vi "Meas_Fast_FID_Bkgnd.vi"(3 "Mode":T5, 5 "Traverse line In":T2 {"Row Duration (mins)" format="%#.1f"; "Row No" min=0; "Trace Gas Concentration (%)" min=0.0 format="%#.2f"; "Emission Rate (l/min)" format="%#.2f"; "Tunnel Speed" format="%#.2f"; "Start X" format="%#.2f"; "Start Y" format="%#.2f"; "Start Z" format="%#.2f"; "End X" format="%#.2f"; "End Y" format="%#.2f"; "End Z" format="%#.2f"; "Averaging time (min)" min=0.0 format="%#.2f"}) -> (0 "Error Message":string, 1 "Status":T1, 2 "Traverse line Out":T2 {"Row Duration (mins)" format="%#.1f"; "Row No" min=0; "Trace Gas Concentration (%)" min=0.0 format="%#.2f"; "Emission Rate (l/min)" format="%#.2f"; "Tunnel Speed" format="%#.2f"; "Start X" format="%#.2f"; "Start Y" format="%#.2f"; "Start Z" format="%#.2f"; "End X" format="%#.2f"; "End Y" format="%#.2f"; "End Z" format="%#.2f"; "Averaging time (min)" min=0.0 format="%#.2f"})   [LabVIEW 2012]
uses:
  Gen Trav/Traverse_cluster.ctl
  Gen Trav/Spacing.ctl
  Controls/Multi_run_mode.ctl
  Controls/User_Specific_mode.ctl
  Gen Trav/Multi_Run_Status.ctl
  Gen Trav/Trav_mode.ctl
  File/Setup_Filetype.ctl
  Controls/Setup.ctl
  Controls/Save_Data.ctl
  Globals/Trav_pos_global.vi
  Globals/Preference_global.vi
panel:
  out "Initial Trav Pos":dbl[](array[numeric]) format="%#.2f"
  # "X           Y            Z"
  # "Start"
  # "End"
  # "X           Y            Z"
  # "Start"
  # "End"
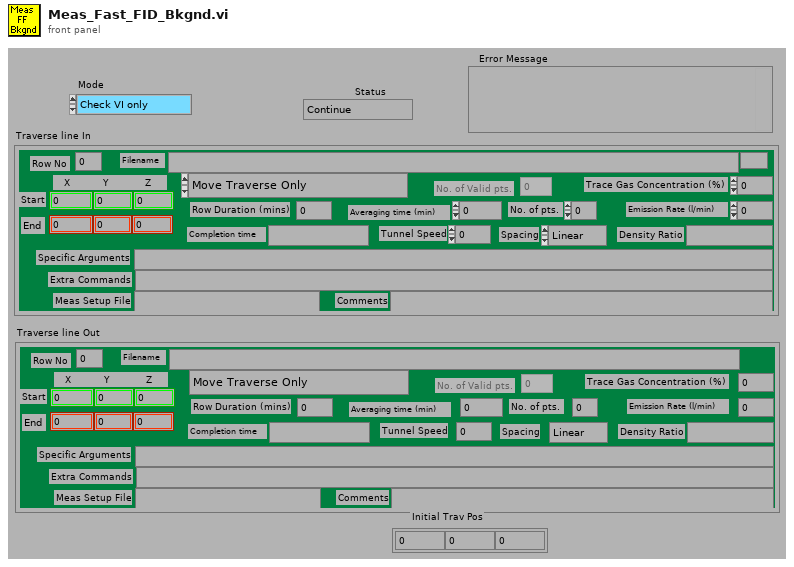
[diagram p1: front panel]
types:
  T1 = typedef "Multi_Run_Status.ctl" = enum16{"Continue", "Jump to Next Point", "Jump to Next Row", "Jump To Fall Back", "Terminate Run"}
  T2 = typedef "Traverse_cluster.ctl" = cluster{"Start X":dbl, "Start Y":dbl, "Start Z":dbl, "End X":dbl, "End Y":dbl, "End Z":dbl, "No. of pts.":i32, "Spacing":T3, "Filename":path, "Tunnel Speed":dbl, "Averaging time (min)":dbl, "Extra Commands":string, "Specific Arguments":string, "Emission Rate (l/min)":dbl, "Trace Gas Concentration (%)":dbl, "Density Ratio":string, "Comments":string, "Row No":i32, "Row Type Selector":T4, "Completion time":string, "Row Duration (mins)":dbl, "No. of Valid pts.":i32, "Meas Setup File":string}
  T3 = typedef "Spacing.ctl" = enum16{"Linear", "Log", "Gauss", "Specified", "N/A"}
  T4 = typedef "Multi_run_mode.ctl" = enum16{"Move Traverse Only", "Set Tunnel Speed Only", "Set Source Only", "Set Measurement Conditions", "Single Measurement", "Vertical Profile", "Lateral Profile", "Longitudinal Profile", "Explore Volume", "Multi-Axis Profile", "Auto Calibrate", "Meas Fast FID Bkgnd", "Check Beam Power", "Scanning Valve Measurement", "Run VI Named:", "Set ADAM Ch", "Wait (minutes)", "Send Message", "Synchronize With:", "Fall Back to this Row", "Turn Off Row Repeating", "Blank Row", "Traverse 3D Volume"}
  T5 = typedef "User_Specific_mode.ctl" = enum16{"Check VI only", "Run VI"}
  T6 = typedef "Tunnel_Coordinates.ctl" = enum16{"Work in Tunnel Coordinates", "Work in Model Coordinates"}
  T7 = typedef "Trav_mode.ctl" = enum16{"Move traverse", "Read traverse position", "Teach Position"}
  T8 = typedef "Setup_Filetype.ctl" = enum16{"Measurement Setups", "Calibration Setups", "General", "Results File Plotter Setups", "Speed Calib Tweaks"}
  T9 = typedef "Save_Data.ctl" = enum16{"Save No Data", "Save Data"}
  T10 = typedef "Setup.ctl" = enum16{"Run Program", "Show Setup", "Save Current Setup", "Setup Front Panel"}
  T11 = typedef "Status_Cluster.ctl" = cluster{"Status":T1, "Error Type":string, "Error Description":string}
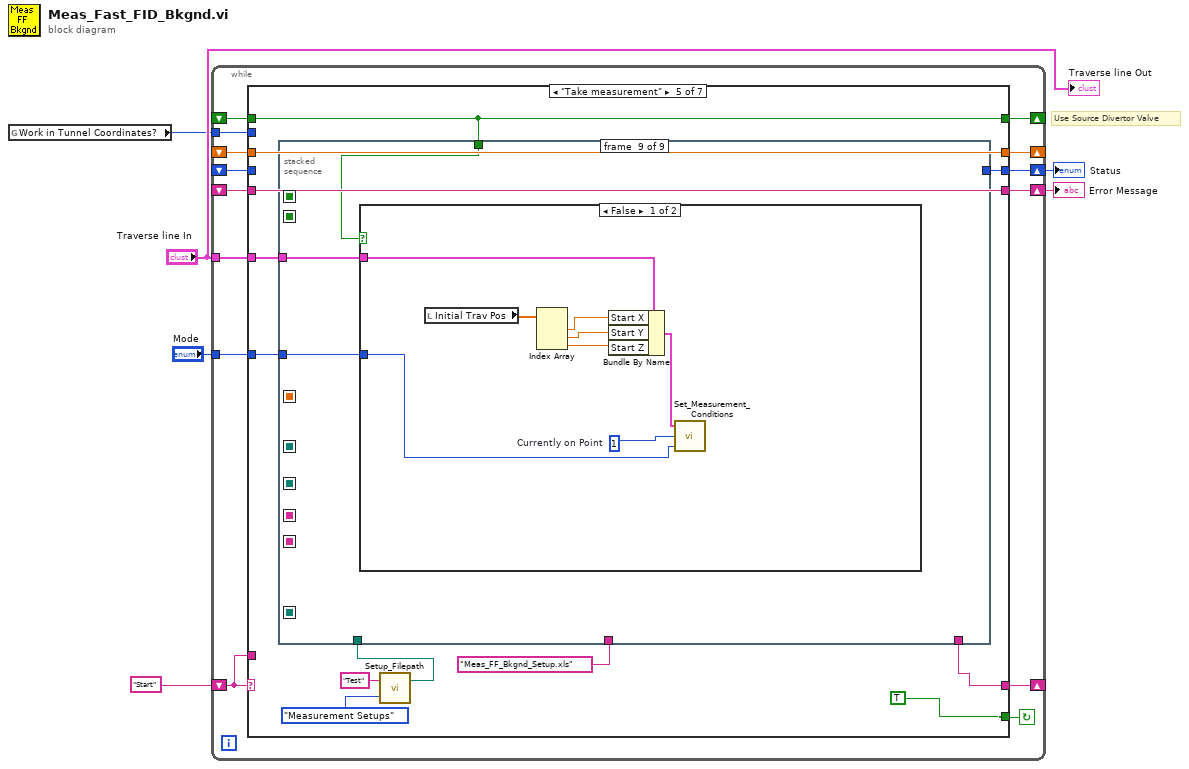
[diagram p0: block diagram]
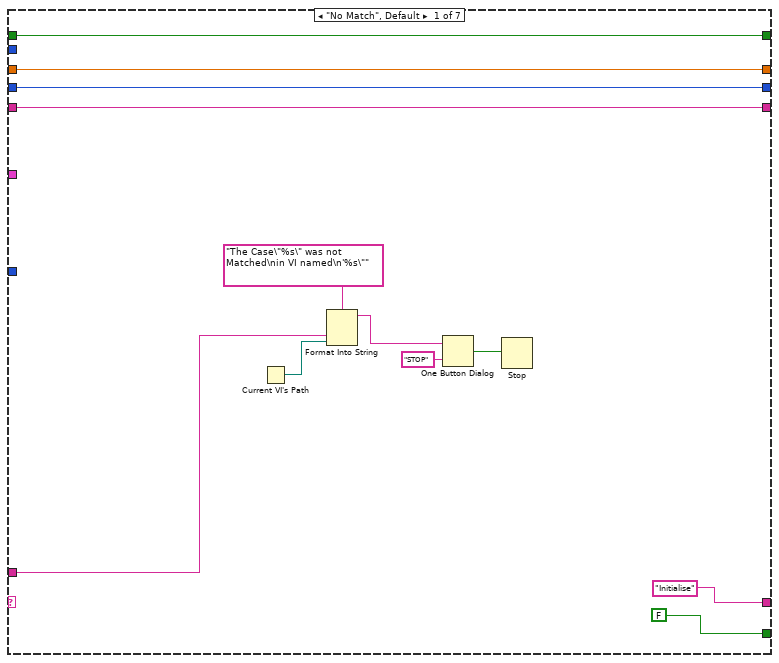
[diagram p2: hidden frame]
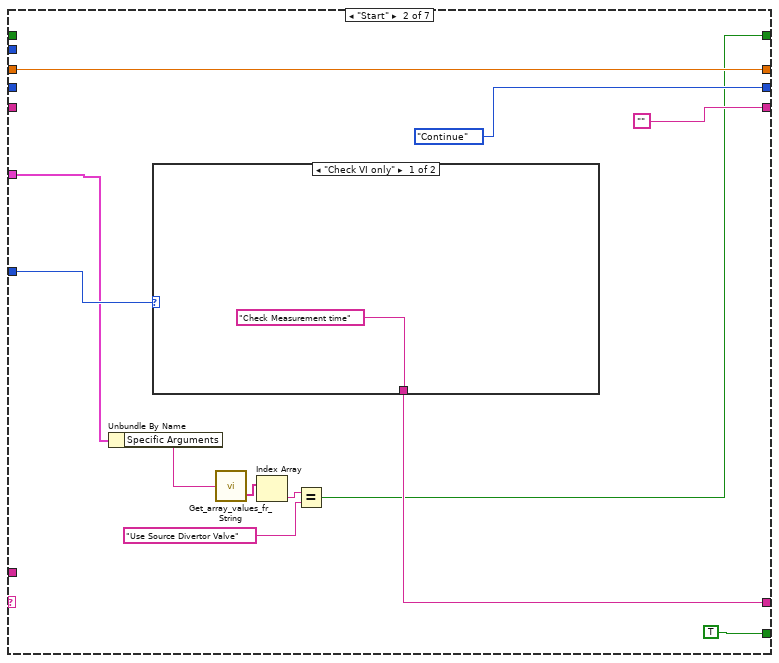
[diagram p3: hidden frame]
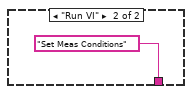
[diagram p4: hidden frame]
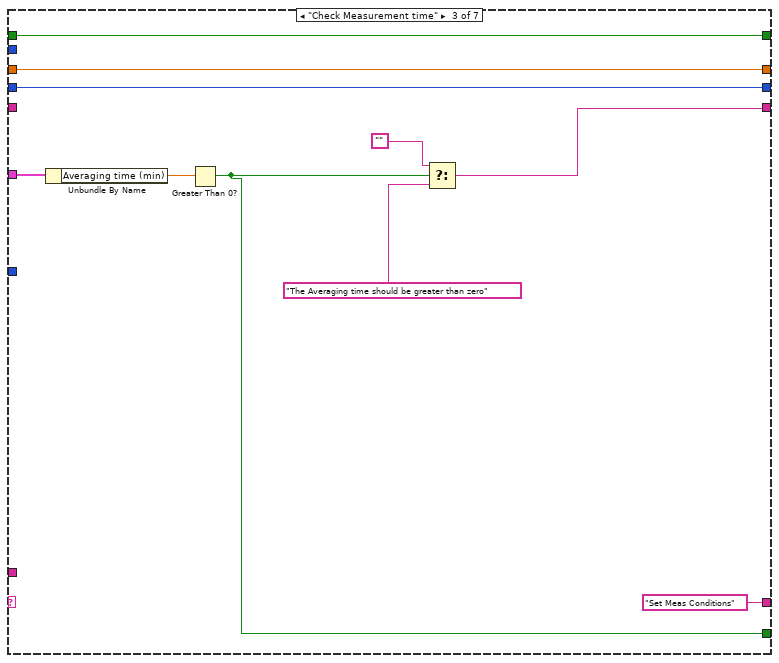
[diagram p5: hidden frame]
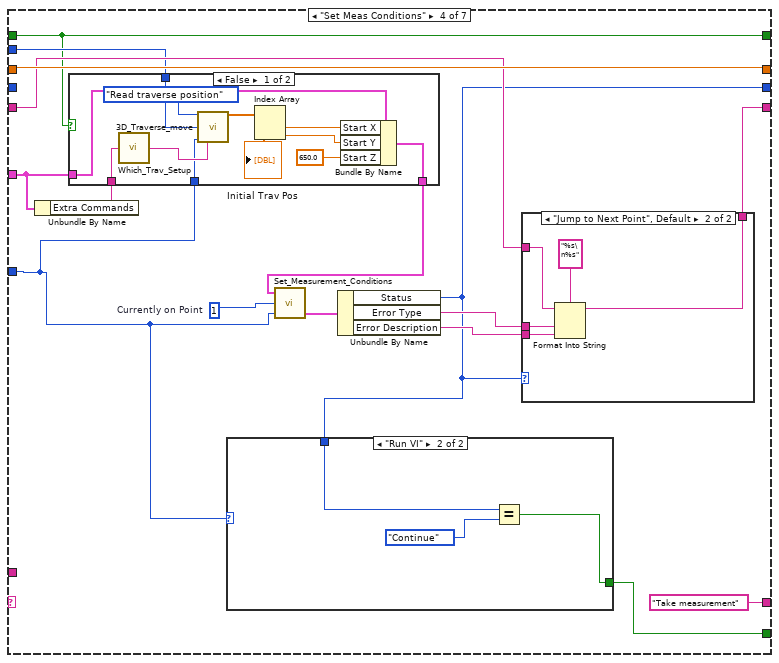
[diagram p6: hidden frame]
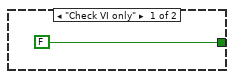
[diagram p9: hidden frame]
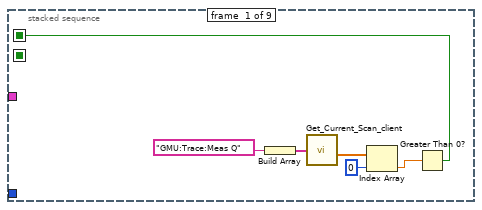
[diagram p10: hidden frame]
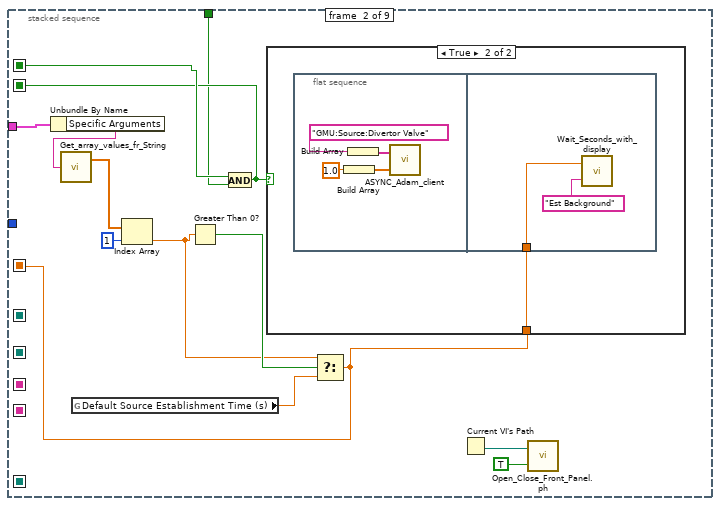
[diagram p11: hidden frame]
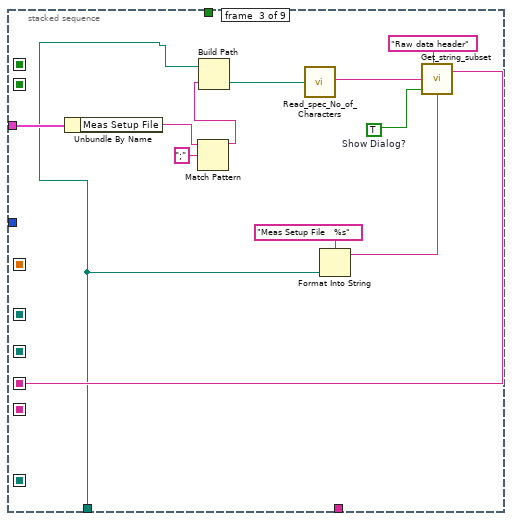
[diagram p13: hidden frame]
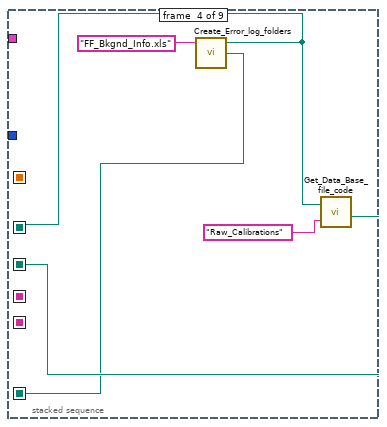
[diagram p14: hidden frame]
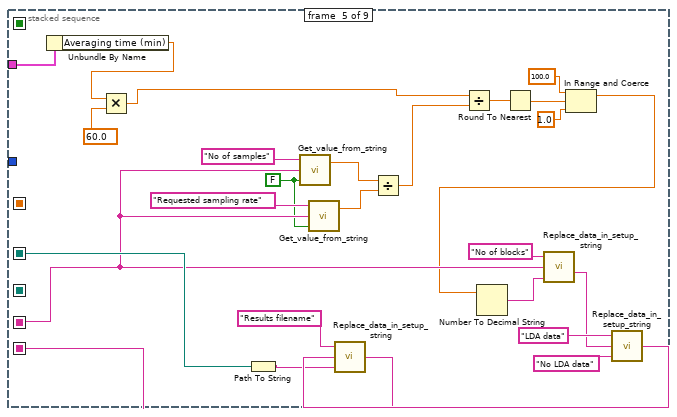
[diagram p15: hidden frame]
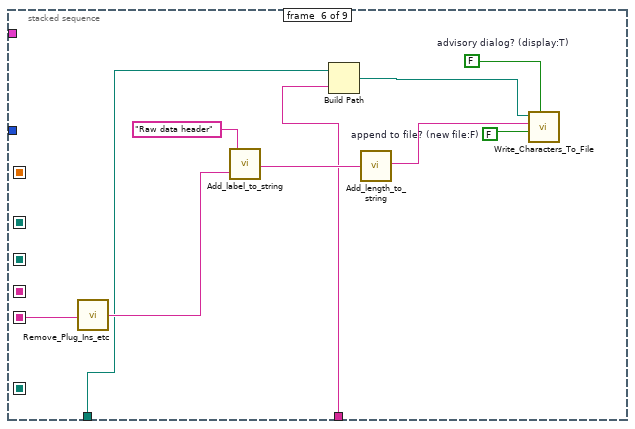
[diagram p16: hidden frame]
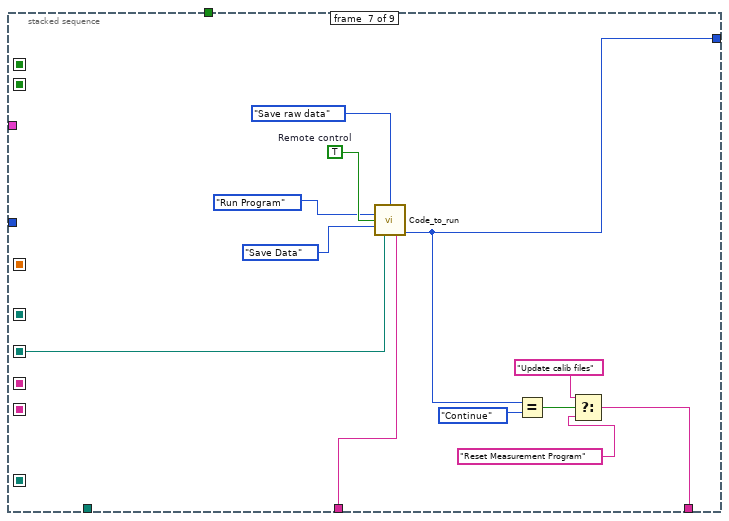
[diagram p17: hidden frame]
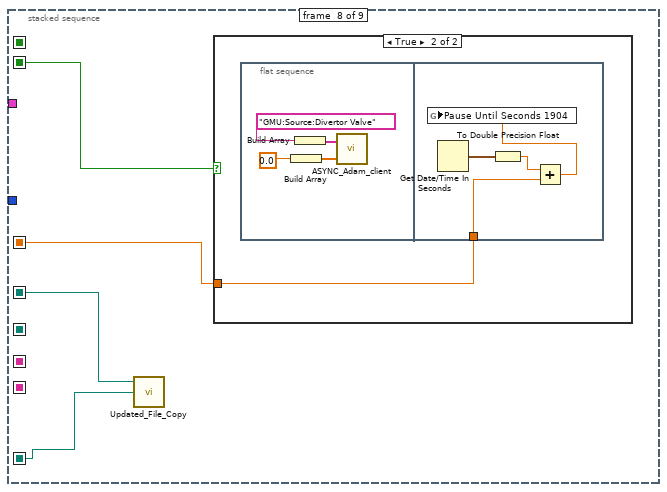
[diagram p18: hidden frame]
diagram:
  # "Use Source Divertor Valve"
  n1 = global read "Trav_pos_global.vi" "Work in Tunnel Coordinates?"() -> (w1:T6)
  n2 = while {
    shift-left: "Start" -> [w18]
    shift-right: [w19] -> _
    shift-right: [w14] -> _
    shift-left: _ -> [w17]
    tunnel: "Mode" -> [w16]
    tunnel: "Traverse line In" -> [w15]
    shift-right: [w13] -> w4
    shift-left: _ -> [w11]
    shift-right: [w12] -> w2
    shift-left: _ -> [w10]
    tunnel: w1 -> [w9]
    shift-right: [w7] -> _
    shift-left: _ -> [w8]
    stop <- w20 continue-if-true
    n3 = case shown="\"Take measurement\"" w18 {
      tunnel: [FALSE TRUE w50 w65 TRUE TRUE FALSE] -> w20
      tunnel: ["Initialise" w42 "Set Meas Conditions" "Take measurement" ("t") w100 "Reset Measurement Program" "End"] -> w19
      tunnel: w18 -> [w27 _ _ _ _ _ _]
      tunnel: w17 -> [w24 w40 w48 w70 w105 w227 _]
      tunnel: w16 -> [_ w43 _ w59 w95 _ _]
      tunnel: w15 -> [_ w36 w56 w61 w103 _ _]
      tunnel: [w24 w40 w48 w70 w105 w227 w232] -> w14
      tunnel: [w23 Multi_Run_Status."Continue" ("Status") w49 w63 w101 w226 w231] -> w13
      tunnel: [w22 "" w52 w66 w104 w225 w234] -> w12
      tunnel: w11 -> [w23 _ w49 _ _ w226 w231]
      tunnel: w10 -> [w22 _ _ w67 w104 w225 w234]
      tunnel: w9 -> [_ _ _ w58 _ _ _]
      tunnel: w8 -> [w21 _ w47 w57 w96 w222 w230]
      tunnel: [w21 w34 w47 w57 w96 w222 w230] -> w7
      frame "No Match", Default {
        n4 = Current VI's Path() -> (path=w26:path)
        n5 = Format Into String(format string="The Case\"%s\" was not Matched\nin VI named\n'%s\"" ("Format String"), w27, w26) -> (resulting string=w30:string)  [unwired: 2 in, 1 out]
        n6 = One Button Dialog(message=w30, button name ("OK")="STOP") -> (true=w28:bool)
        n7 = Stop(stop? (T)=w28) -> ()
      }
      frame "Start" {
        n8 = Unbundle By Name(w36) -> ("Specific Arguments"=w35:string)
        n9 = case shown="\"Check VI only\"" w43 {
          tunnel: ["Check Measurement time" "Set Meas Conditions"] -> w42
          frame "Check VI only" {
          }
          frame "Run VI" {
          }
        }
        n10 = call "Get_array_values_fr_String.vi"("String Value"=w35) -> ("String array"=w38:string[])  [unwired: 1 out]
        n11 = Index Array(array=w38) -> (element=w37:string)  [unwired: 1 in]
        n12 = Equal?(x=w37, y="Use Source Divertor Valve") -> (x = y?=w34:bool)
      }
      frame "Check Measurement time" {
        n13 = Unbundle By Name(w56) -> ("Averaging time (min)"=w55:dbl)
        n14 = Greater Than 0?(x=w55) -> (x > 0?=w50:bool)
        n15 = Select(t="", s=w50, f="The Averaging time should be greater than zero") -> (s? t:f=w52:string)
      }
      frame "Set Meas Conditions" {
        w72 = 1  # Currently on Point
        n16 = Unbundle By Name(w61) -> ("Extra Commands"=w60:string)
        n17 = case shown="False" w57 {
          tunnel: [w83 w84] -> w62
          tunnel: w61 -> [w82 w84]
          tunnel: w60 -> [w81 _]
          tunnel: w59 -> [w79 _]
          tunnel: w58 -> [w78 _]
          frame False {
            n18 = call "Which_Trav_Setup.vi"("Extra Command String"=w81) -> ("Traverse Setup"=w80:string)
            n19 = call "3D_Traverse_move.vi"("Mode"=Trav_mode."Read traverse position", "Work in Tunnel Coordinates"=w78, "Simulate/Run"=w79, "Traverse name"=w80) -> ("Trav Position achieved"=w74:dbl[])  [unwired: 5 in, 6 out]
            "Initial Trav Pos" <- w74
            n20 = Index Array(array=w74) -> (element #1=w76:dbl, element #2=w73:dbl)  [unwired: 2 in]
            n21 = Bundle By Name(cluster=w82, "Start X"=w76, "Start Y"=w73, "Start Z"=650.0) -> (w83:T2)
          }
          frame True {
          }
        }
        n22 = call "Set_Measurement_Conditions.vi"("Simulate/Run"=w59, "Currently on Point"=w72, "Traverse line"=w62) -> ("Status Cluster"=w71:T11)  [unwired: 2 out]
        n23 = Unbundle By Name(w71) -> ("Status"=w63:T1, "Error Type"=w69:string, "Error Description"=w68:string)
        n24 = case shown="\"Run VI\"" w59 {
          tunnel: [FALSE w93] -> w65
          tunnel: w63 -> [_ w94]
          frame "Check VI only" {
          }
          frame "Run VI" {
            n25 = Equal?(x=w94, y=Multi_Run_Status."Continue" ("Status")) -> (x = y?=w93:bool)
          }
        }
        n26 = case shown="\"Jump to Next Point\", Default" w63 {
          tunnel: w69 -> [_ w90]
          tunnel: w68 -> [_ w89]
          tunnel: w67 -> [w85 w88]
          tunnel: [w85 w87] -> w66
          frame "Continue" {
          }
          frame "Jump to Next Point", Default {
            n27 = Format Into String(format string="%s\n%s", initial string=w88, w90, w89) -> (resulting string=w87:string)  [unwired: 1 in, 1 out]
          }
        }
      }
      frame "Take measurement" {
        n28 = call "Setup_Filepath.vi"("Setup File Type"=Setup_Filetype."Measurement Setups", "Filename in"="Test") -> ("Directory"=w97:path)  [unwired: 1 out]
        n29 = stacked-sequence {
          seq-local: [_ _ w142 _ _ _ _ _ _] -> [_ _ _ _ w157 _ _ _ _]
          seq-local: [_ _ _ _ w166 _ _ _ _] -> [_ _ _ _ _ w178 _ _ _]
          seq-local: [_ _ _ w146 _ _ _ _ _] -> [_ _ _ _ _ _ w193 _ _]
          seq-local: [_ _ _ w148 _ _ _ _ _] -> [_ _ _ _ w165 _ _ w201 _]
          seq-local: [_ w114 _ _ _ _ _ _ _] -> [_ _ _ _ _ _ _ w199 _]
          seq-local: [_ w116 _ _ _ _ _ _ _] -> [_ _ _ _ _ _ _ w198 _]
          seq-local: [_ _ _ w145 _ _ _ _ _] -> [_ _ _ _ _ _ _ w200 _]
          seq-local: [w107 _ _ _ _ _ _ _ _] -> [_ w115 _ _ _ _ _ _ _]
          tunnel: "Meas_FF_Bkgnd_Setup.xls" -> [_ _ _ _ _ w180 w195 _ _]
          tunnel: w103 -> [_ w123 w139 _ w161 _ _ _ w213]
          tunnel: [_ _ _ _ _ _ w191 _ _] -> w101
          tunnel: [_ _ _ _ _ _ w188 _ _] -> w100
          tunnel: w97 -> [_ _ w134 _ _ w176 _ _ _]
          tunnel: w96 -> [_ w113 _ _ _ _ _ _ w211]
          tunnel: w95 -> [_ _ _ _ _ _ _ _ w212]
          frame #0 {
            n30 = Build Array("GMU:Trace:Meas Q") -> (w111:string[])
            n31 = call "Get_Current_Scan_client.vi"("ADAM Ch Names"=w111) -> ("Numerical Values"=w109:dbl[])  [unwired: 3 out]
            n32 = Index Array(array=w109, index=0) -> (element=w108:dbl)
            n33 = Greater Than 0?(x=w108) -> (x > 0?=w107:bool)
          }
          frame #1 {
            n34 = Unbundle By Name(w123) -> ("Specific Arguments"=w122:string)
            n35 = call "Get_array_values_fr_String.vi"("String Value"=w122) -> ("Numeric Array"=w120:dbl[])  [unwired: 1 out]
            n36 = global read "Preference_global.vi" "Default Source Establishment Time (s)"() -> (w117:dbl)
            n37 = Index Array(array=w120, index=1) -> (element=w118:dbl)
            n38 = Greater Than 0?(x=w118) -> (x > 0?=w119:bool)
            n39 = And(x=w115, y=w113) -> (x .and. y?=w114:bool)
            n40 = Select(t=w118, s=w119, f=w117) -> (s? t:f=w116:dbl)
            n41 = case shown="True" w114 {
              tunnel: w116 -> [_ w126]
              frame False {
              }
              frame True {
                n42 = flat-sequence {
                  tunnel: w126 -> [w131]
                  frame #0 {
                    n43 = Build Array(1.0) -> (w127:dbl[])
                    n44 = Build Array("GMU:Source:Divertor Valve") -> (w128:string[])
                    n45 = call "ASYNC_Adam_client.vi"("Values"=w127, "Channel Names"=w128) -> ()  [unwired: 2 out]
                  }
                  frame #1 {
                    n46 = call "Wait_Seconds_with_display.vi"("Message"="Est Background", "Seconds to wait"=w131) -> ()  [unwired: 2 out]
                  }
                }
              }
            }
            n47 = Current VI's Path() -> (path=w124:path)
            n48 = call "Open_Close_Front_Panel.ph.vi"("Front Panel Window:Open"=TRUE, "VI path"=w124) -> ()  [unwired: 2 out]
          }
          frame #2 {
            w140 = TRUE  # Show Dialog?
            n49 = Unbundle By Name(w139) -> ("Meas Setup File"=w137:string)
            n50 = Match Pattern(string=w137, regular expression=";") -> (before substring=w136:string)  [unwired: 4 out]
            n51 = Build Path(base path=w134, name or relative path=w136) -> (appended path=w141:path)
            n52 = call "Read_spec_No_of_Characters.vi"("Filename"=w141) -> ("character string"=w143:string)  [unwired: 1 out]
            n53 = Format Into String(format string="Meas Setup File   %s", w134) -> (resulting string=w133:string)  [unwired: 2 in, 1 out]
            n54 = call "Get_string_subset.vi"("String Name"=w133, "Show Dialog?"=w140, "String to split"=w143, "File Label"="Raw data header") -> ("Output string"=w142:string)  [unwired: 1 out]
          }
          frame #3 {
            n55 = call "Create_Error_log_folders.vi"("Log Filename"="FF_Bkgnd_Info.xls") -> ("Server copy Location"=w145:path, "Local Log File"=w148:path)  [unwired: 2 in, 1 out]
            n56 = call "Get_Data_Base_file_code.vi"("Results Filename"=w148, "Data Type"="Raw_Calibrations") -> ("Raw Data File Name"=w146:path)  [unwired: 3 out]
          }
          frame #4 {
            w154 = FALSE ("Show Dialog?")
            n57 = Unbundle By Name(w161) -> ("Averaging time (min)"=w160:dbl)
            n58 = Multiply(x=w160, y=60.0) -> (x*y=w162:dbl)
            n59 = Path To String(path=w165) -> (string=w164:string)
            n60 = call "Get_value_from_string.vi"("Show Dialog?"=w154, "Input string"=w157, "Variable name"="No of samples") -> ("Value"=w155:dbl)  [unwired: 1 out]
            n61 = call "Get_value_from_string.vi"("Show Dialog?"=w154, "Input string"=w157, "Variable name"="Requested sampling rate") -> ("Value"=w156:dbl)  [unwired: 1 out]
            n62 = Divide(x=w155, y=w156) -> (x/y=w175:dbl)
            n63 = Divide(x=w162, y=w175) -> (x/y=w174:dbl)
            n64 = Round To Nearest(number=w174) -> (nearest integer value=w153:dbl)
            n65 = In Range and Coerce(upper limit=100.0, x=w153, lower limit=1.0) -> (coerced(x)=w150:dbl)  [unwired: 1 out]
            n66 = Number To Decimal String(number=w150) -> (decimal integer string=w172:string)  [unwired: 1 out]
            n67 = call "Replace_data_in_setup_string.vi"("New data string"=w172, "Input string"=w157, "Variable name"="No of blocks") -> ("Appended string"=w169:string)
            n68 = call "Replace_data_in_setup_string.vi"("New data string"="No LDA data", "Input string"=w169, "Variable name"="LDA data" ("Label for characters")) -> ("Appended string"=w167:string)
            n69 = call "Replace_data_in_setup_string.vi"("New data string"=w164, "Input string"=w167, "Variable name"="Results filename") -> ("Appended string"=w166:string)
          }
          frame #5 {
            w184 = FALSE  # advisory dialog? (display:T)
            w185 = FALSE  # append to file? (new file:F)
            n70 = call "Remove_Plug_Ins_etc.vi"("Input String"=w178) -> ("Output string"=w177:string)
            n71 = call "Add_label_to_string.vi"("String to write"=w177, "File Label"="Raw data header") -> ("Output string"=w181:string)
            n72 = Build Path(base path=w176, name or relative path=w180) -> (appended path=w179:path)
            n73 = call "Add_length_to_string.vi"("String in"=w181) -> ("String out"=w183:string)
            n74 = call "Write_Characters_To_File.vi"("file path (dialog if empty)"=w179, "advisory dialog? (display:T)"=w184, "character string"=w183, "append to file? (new file:F)"=w185) -> ()  [unwired: 1 in, 4 out]
          }
          frame #6 {
            w197 = TRUE  # Remote control
            n75 = call "Code_to_run.vi"("Raw data option"=enum16{"Save raw data", "Raw data not saved"}."Save raw data", "setup"=Setup."Run Program", "Remote control"=w197, "File"=Save_Data."Save Data", "Raw data file"=w193, "Setup filename"=w195) -> ("Status"=w191:T1)  [unwired: 5 in, 4 out]
            n76 = Equal?(x=w191, y=Multi_Run_Status."Continue" ("Status")) -> (x = y?=w189:bool)
            n77 = Select(t="Update calib files", s=w189, f="Reset Measurement Program") -> (s? t:f=w188:string)
          }
          frame #7 {
            n78 = call "Updated_File_Copy.vi"("Target Path"=w200, "Source Path"=w201) -> ()  [unwired: 2 out]
            n79 = case shown="True" w199 {
              tunnel: w198 -> [_ w202]
              frame False {
              }
              frame True {
                n80 = flat-sequence {
                  tunnel: w202 -> [w208]
                  frame #0 {
                    n81 = Build Array(0.0) -> (w203:dbl[])
                    n82 = Build Array("GMU:Source:Divertor Valve") -> (w204:string[])
                    n83 = call "ASYNC_Adam_client.vi"("Values"=w203, "Channel Names"=w204) -> ()  [unwired: 2 out]
                  }
                  frame #1 {
                    n84 = Get Date/Time In Seconds() -> (seconds since 1Jan1904=w210:timestamp)
                    n85 = To Double Precision Float(number=w210) -> (double precision float=w209:dbl)
                    n86 = Add(x=w209, y=w208) -> (x+y=w207:dbl)
                    n87 = global write "Trav_pos_global.vi" "Pause Until Seconds 1904"(w207) -> ()
                  }
                }
              }
            }
          }
          frame #8 {
            n88 = case shown="False" w211 {
              tunnel: w213 -> [w216 _]
              tunnel: w212 -> [w214 _]
              frame False {
                w221 = 1  # Currently on Point
                n89 = local read "Initial Trav Pos"() -> (w220:dbl[])
                n90 = Index Array(array=w220) -> (element #1=w219:dbl, element #2=w218:dbl, element #3=w217:dbl)  [unwired: 3 in]
                n91 = Bundle By Name(cluster=w216, "Start X"=w219, "Start Y"=w218, "Start Z"=w217) -> (w215:T2)
                n92 = call "Set_Measurement_Conditions.vi"("Simulate/Run"=w214, "Currently on Point"=w221, "Traverse line"=w215) -> ()  [unwired: 3 out]
              }
              frame True {
              }
            }
          }
        }
      }
      frame "Update calib files" {
        w223 = dbl[] [] ("C (ppm)")
        w224 = TRUE  # Specific Bkgnd Meas?
        n93 = call "Update_FFID_Bkgnd_info.vi"("Specific Bkgnd Meas?"=w224, "c^2 (ppm^2)"=w223, "C (ppm)"=w223) -> ()  [unwired: 1 in]
      }
      frame "Reset Measurement Program" {
        n94 = Get Date/Time In Seconds() -> (seconds since 1Jan1904=w233:timestamp)
        n95 = To Double Precision Float(number=w233) -> (double precision float=w232:dbl)
      }
    }
  }
  "Error Message" <- w2
  "Status" <- w4
  "Traverse line Out" <- "Traverse line In"
